vi "Exp_ICCD_SetSequentialEndingGateProperties.vi"(8 "error in (no error)":errorcluster, 9 "Sequential Ending Gate Width (ns)":dbl, 10 "Sequential Ending Gate Delay (ns)":dbl, 11 "LightField Automation in":refnum<class "LightField Automation.lvclass">) -> (0 "error out":errorcluster, 3 "LightField Automation out":refnum<class "LightField Automation.lvclass">)   [LabVIEW 2020, in "LightField Automation.lvclass"]
uses:
  LightField Automation.lvclass
  C:/Program Files/Princeton Instruments/LightField/AddInViews/PrincetonInstruments.LightFieldViewV3.dll
  C:/Program Files/Princeton Instruments/LightField/PrincetonInstruments.LightFieldAddInSupportServices.dll
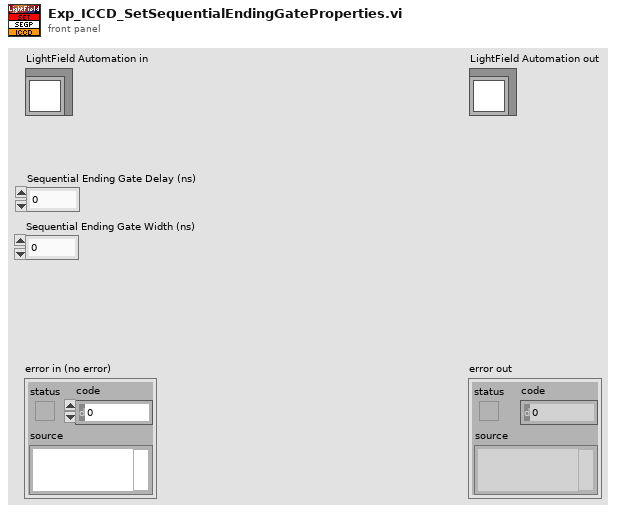
[diagram p1: front panel]
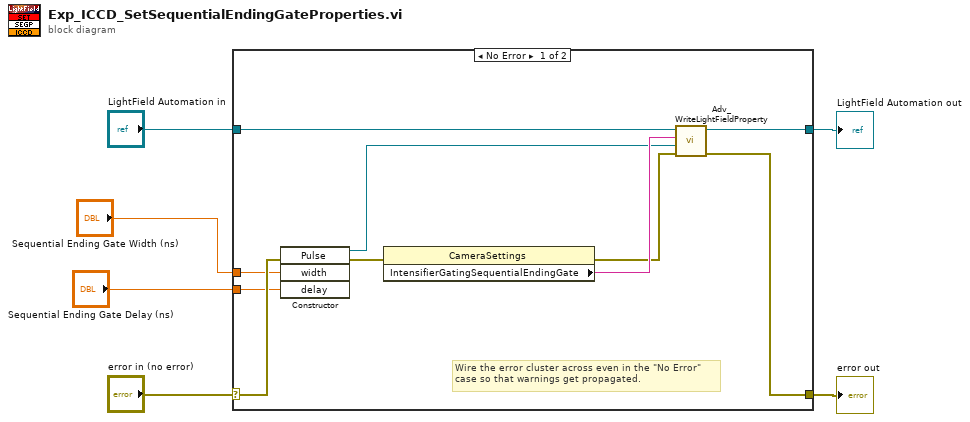
[diagram p0: block diagram]
diagram:
  n1 = case shown="No Error" "error in (no error)" {
    selector: "error in (no error)" -> [w16 w18]
    tunnel: [w7 w18] -> w5
    tunnel: [w12 w17] -> w3
    tunnel: "LightField Automation in" -> [w11 w17]
    tunnel: "Sequential Ending Gate Width (ns)" -> [w14 _]
    tunnel: "Sequential Ending Gate Delay (ns)" -> [w13 _]
    frame No Error {
      # "Wire the error cluster across even in the \"No Error\"\ncase so that warnings get propagated."
      n2 = constructor class="Pulse"(error in=w16, "width"=w14, "delay"=w13) -> (reference out=w8:refnum<k24>, error out=w15:errorcluster)  [unwired: 2 in, 3 out]
      n3 = property class="CameraSettings"(error in=w15) -> (error out=w9:errorcluster, "IntensifierGatingSequentialEndingGate"=w10:string)  [unwired: 1 in, 1 out]
      n4 = call "Adv_WriteLightFieldProperty.vi"("error in (no error)"=w9, "value"=w8, "setting"=w10, "LightField Automation in"=w11) -> ("error out"=w7:errorcluster, "LightField Automation out"=w12:refnum<class "LightField Automation.lvclass">)  [unwired: 6 in]
    }
    frame Error {
    }
  }
  "error out" <- w5
  "LightField Automation out" <- w3
